vi "Read_delimityef.vi"() -> ()   [LabVIEW 2022 SP3]
uses:
  <vilib>/Utility/file.llb/Read Delimited Spreadsheet (string).vi
panel:
  out "Array":cluster{dbl, string}[](array[cluster])
  in  "OK Button":bool
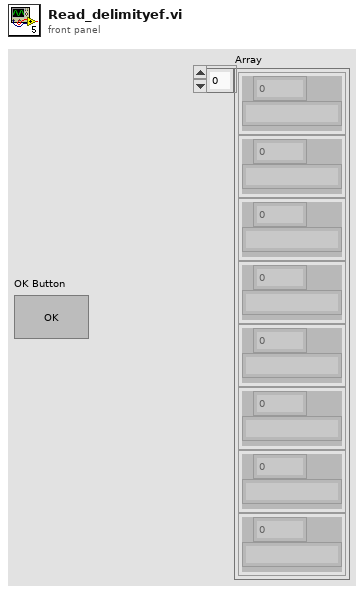
[diagram p1: front panel]
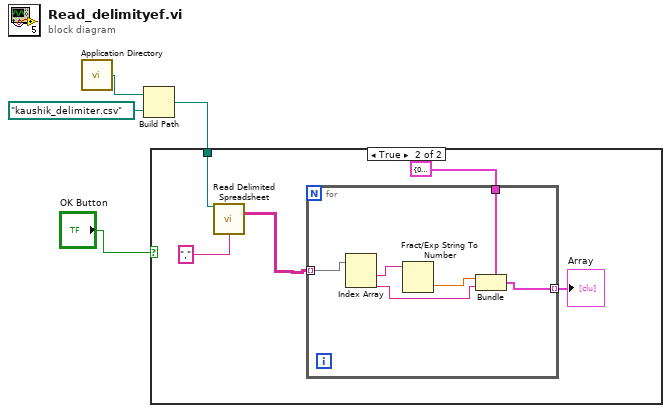
[diagram p0: block diagram]
diagram:
  n1 = call <vilib>:"Application Directory.vi"() -> ("Application Directory"=w4:path)
  n2 = Build Path(base path=w4, name or relative path=path "kaushik_delimiter.csv") -> (appended path=w1:path)
  n3 = case shown="True" "OK Button" {
    tunnel: w1 -> [_ w9]
    frame False {
    }
    frame True {
      n4 = call-poly <vilib>:"Read Delimited Spreadsheet.vi"("file path (dialog if empty)"=w9, "delimiter (\\t)"="," ("delimiter (\\t)")) -> ("all rows"=w7:string[][])  [unwired: 8 in, 5 out]
      n5 = for {
        tunnel: w7 -> [w15] mode=indexing
        tunnel: cluster{dbl, string} {0.0, ""} -> [w11]
        tunnel: [w10] -> w5 mode=indexing
        n6 = Index Array(array=w15) -> (element #1=w14:string, element #2=w12:string)  [unwired: 2 in]
        n7 = Fract/Exp String To Number(string=w14) -> (number=w13:dbl)  [unwired: 3 in, 1 out]
        n8 = Bundle(cluster=w11, w13, w12) -> (w10:cluster{dbl, string})
      }
      "Array" <- w5
    }
  }
